vi "Calculate Constants.vi"(1 "Z":dbl, 2 "Y":dbl, 3 "X":dbl) -> (0 "constants cluster":cluster{"a":dbl, "b":dbl, "c":dbl, "d":dbl})   [LabVIEW 2016]
panel:
  in  "constant":dbl=1.0
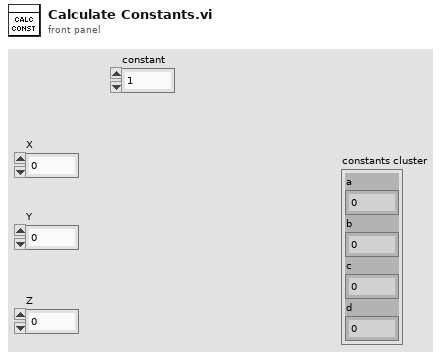
[diagram p1: front panel]
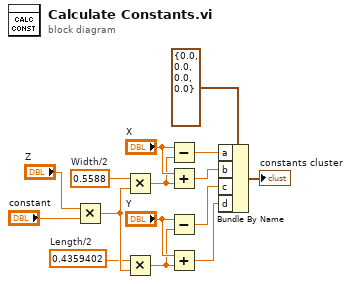
[diagram p0: block diagram]
diagram:
  w6 = 0.4359402  # Length/2
  w9 = 0.5588  # Width/2
  n1 = Multiply(x="Z", y="constant") -> (x*y=w7:dbl)
  n2 = Multiply(x=w9, y=w7) -> (x*y=w1:dbl)
  n3 = Multiply(x=w6, y=w7) -> (x*y=w3:dbl)
  n4 = Subtract(x="X", y=w1) -> (x-y=w11:dbl)
  n5 = Add(x="X", y=w1) -> (x+y=w8:dbl)
  n6 = Subtract(x="Y", y=w3) -> (x-y=w5:dbl)
  n7 = Add(x="Y", y=w3) -> (x+y=w2:dbl)
  n8 = Bundle By Name(cluster=cluster{"a":dbl, "b":dbl, "c":dbl, "d":dbl} {"a"=0.0, "b"=0.0, "c"=0.0, "d"=0.0}, "a"=w11, "b"=w8, "c"=w5, "d"=w2) -> (→"constants cluster":cluster{"a":dbl, "b":dbl, "c":dbl, "d":dbl})
